vi "LabVIEW Interface MAIN QMH.vi"() -> ()   [LabVIEW 2018]
uses:
  src/geve-serial_config_cluster.ctl
panel:
  out "title":string
  out "Motor Position":dbl
  out "Plateau Pressure":dbl
  out "Pressure":dbl
  out "title1":string="LIVE DATA"
  out "Mixed Signal Graph":T1(graph)
  out "BPM":dbl
  out "PEEP":dbl
  out "Tidal Volume":dbl
  out "IE Ratio":dbl
  out "title 2":string="LIVE DATA"
  out "log":string
  out "INITIALISATION ERROR":bool
  out "HIGH PRESSURE":bool
  out "LOW PRESSURE":bool
  # "LATEST VALUE"
  # "Motor Position"
  # "Plateau Pressure"
  # "Pressure"
  # "POTENTIOMETERS SETTINGS"
  # "BPM"
  # "PEEP"
  # "IE RATIO"
  # "TIDAL VOLUME"
  # "ALARMS"
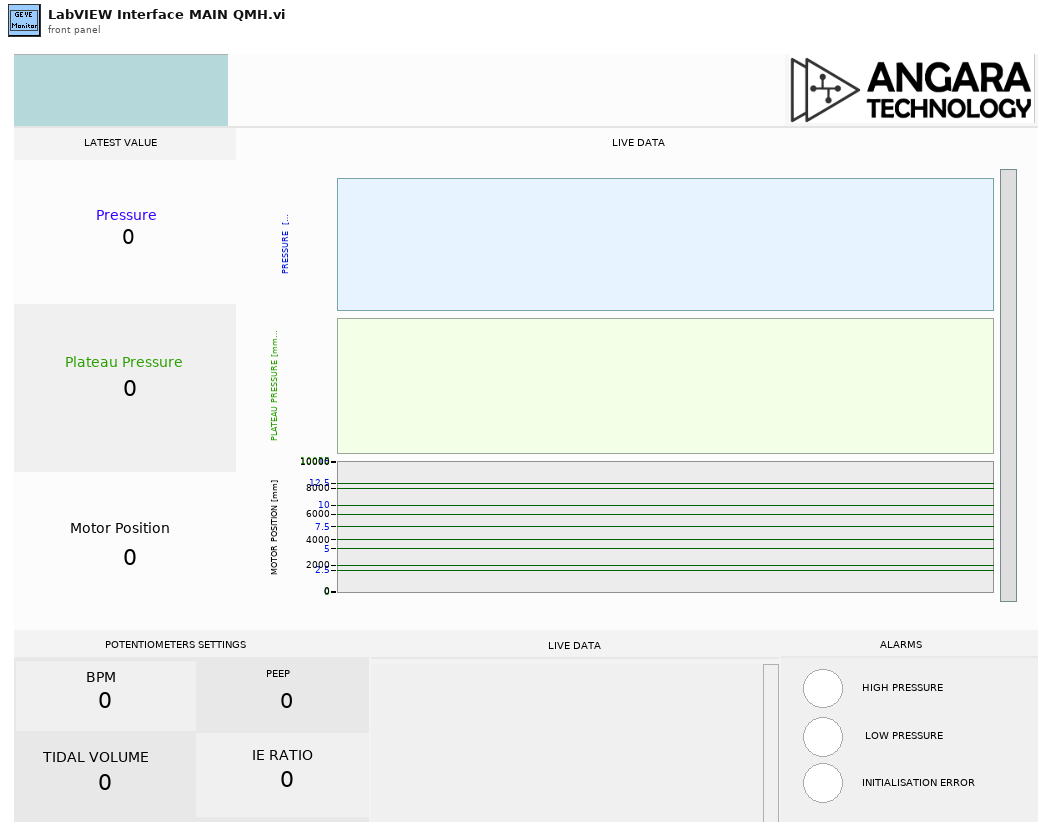
[diagram p1: front panel]
types:
  T1 = cluster{"Time Stamp Array":timestamp[], "Time Stamp Array":dbl[]}[]
  T2 = typedef "geve-runtime_data_cluster.ctl" = cluster{"GEVE Ventilator Monitoring Data":T3, "Serial Port Configuration":T4, "Serial Read Return Count":u32, "Read Buffer":string, "Communication Timeout?":bool, "com-refs":T5}
  T3 = typedef "geve-monitoring_data_cluster.ctl" = cluster{"On/Off":bool, "Error Ack":bool, "bpm":dbl, "VT":dbl, "IE":dbl, "PEEP":dbl, "Pressure":dbl, "Plateau Pressure":dbl, "Motor Position":dbl, "Alarm P High":bool, "Alarm P Low":bool, "Alarm Init":bool}
  T4 = typedef "geve-serial_config_cluster.ctl" = cluster{"timeout (ms)":u32, "VISA resource name":refnum<visa-resource-name>, "baud rate":u32, "max expected byte count":u32}
  T5 = typedef "geve-com_ref_cluster.ctl" = cluster{"msg-self Q":refnum<queue>, "gui stop event":refnum<user-event>}
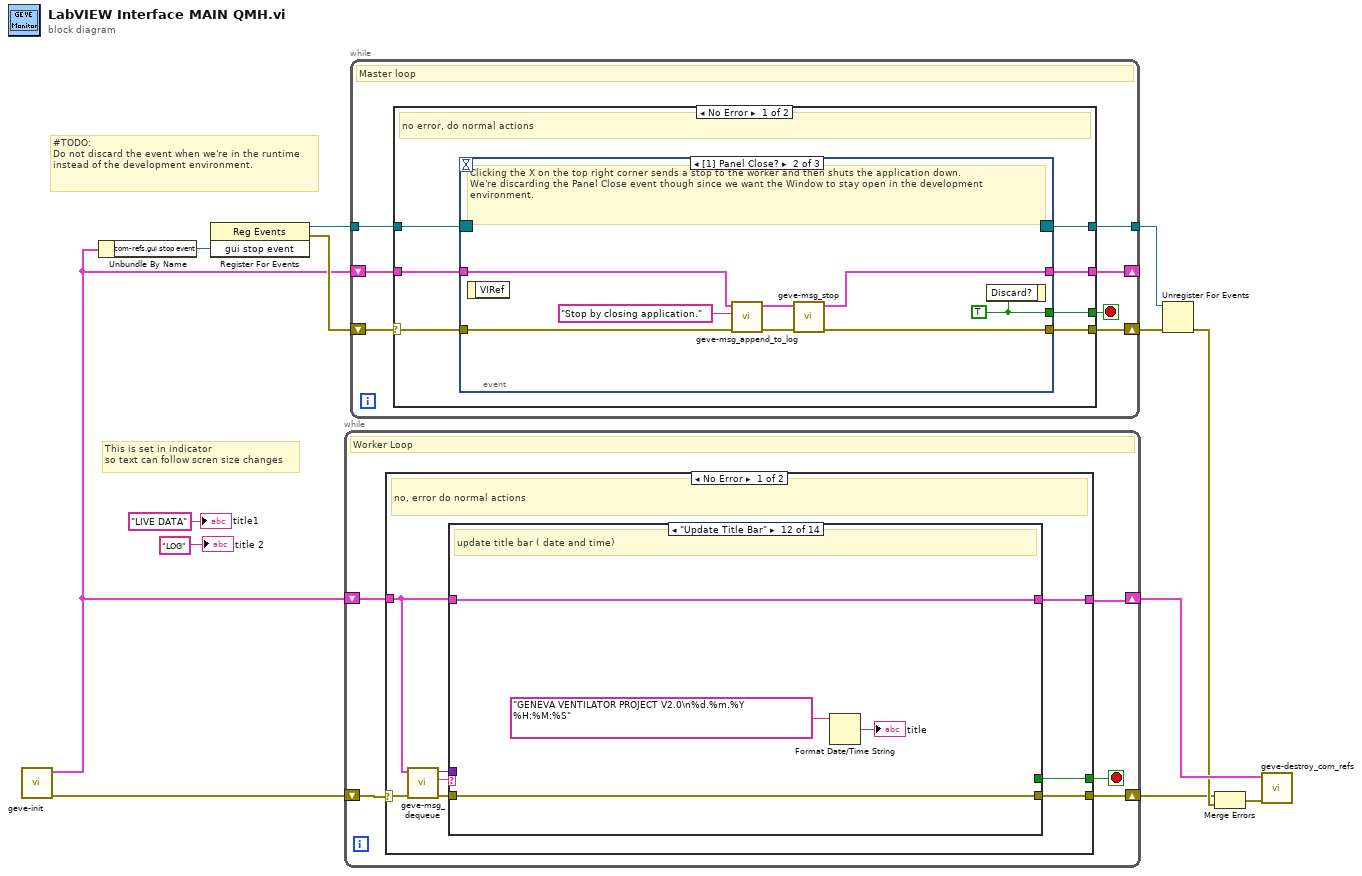
[diagram p0: block diagram]
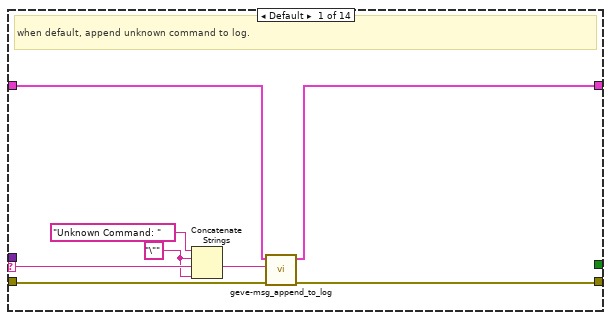
[diagram p2: hidden frame]
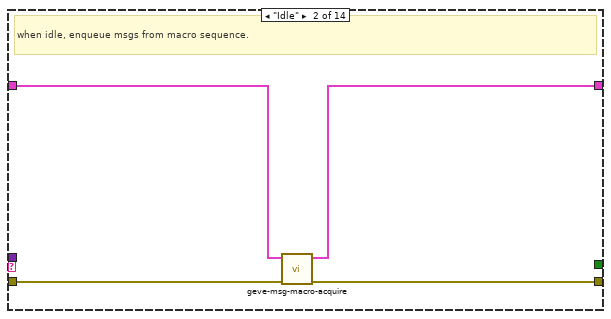
[diagram p3: hidden frame]
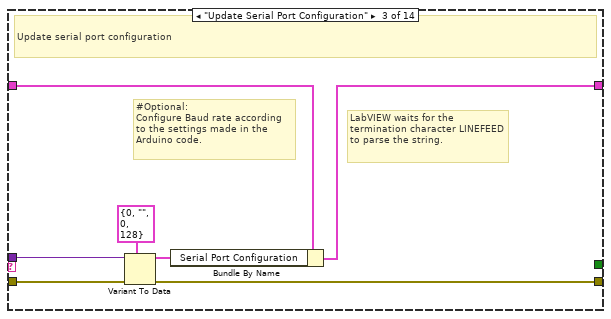
[diagram p4: hidden frame]
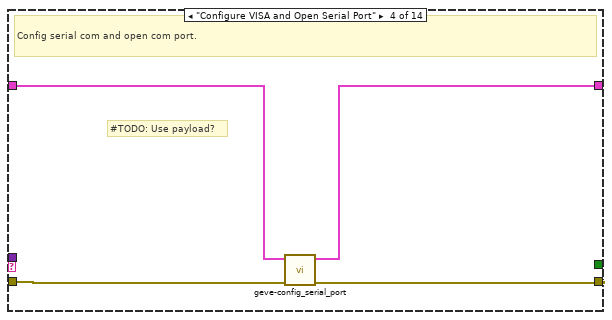
[diagram p5: hidden frame]
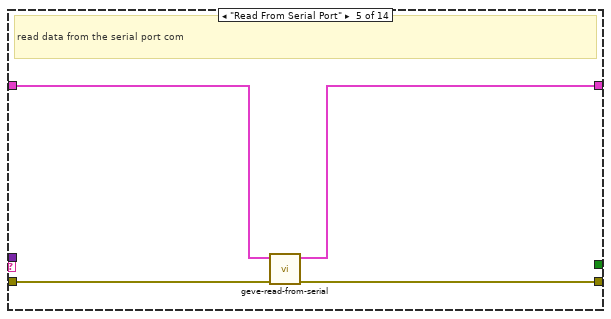
[diagram p6: hidden frame]
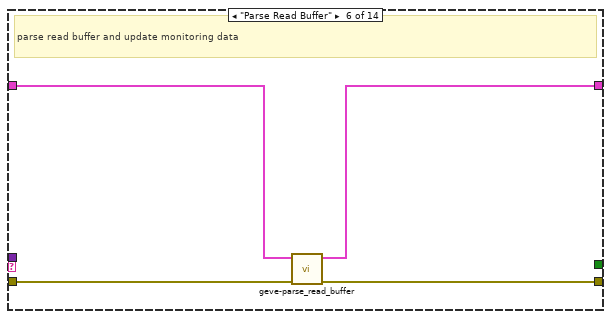
[diagram p7: hidden frame]
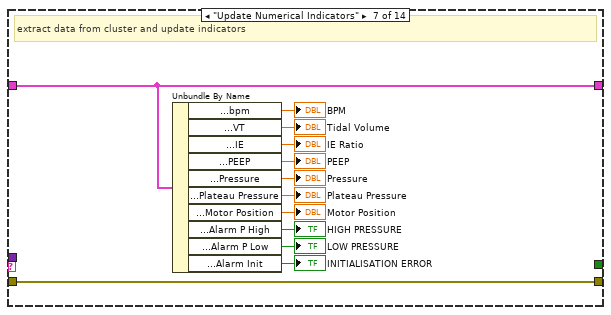
[diagram p8: hidden frame]
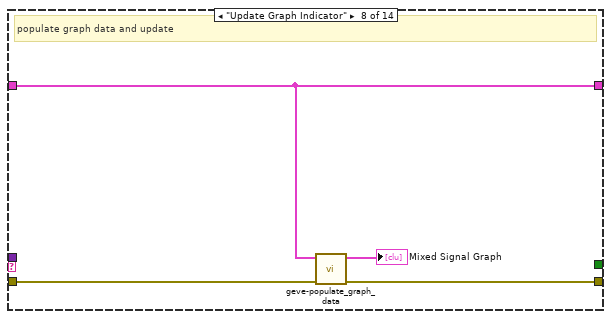
[diagram p9: hidden frame]
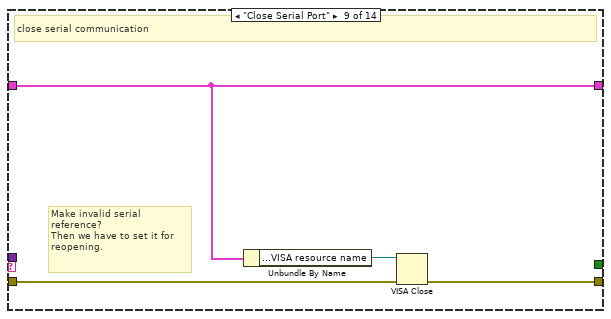
[diagram p10: hidden frame]
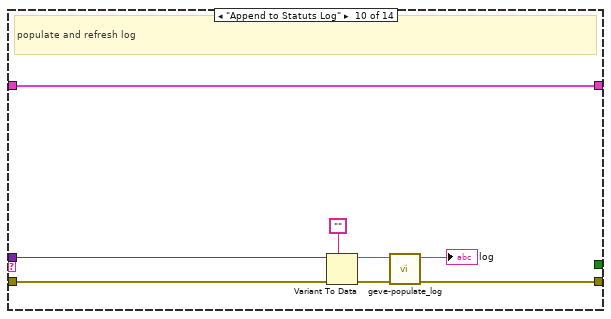
[diagram p11: hidden frame]
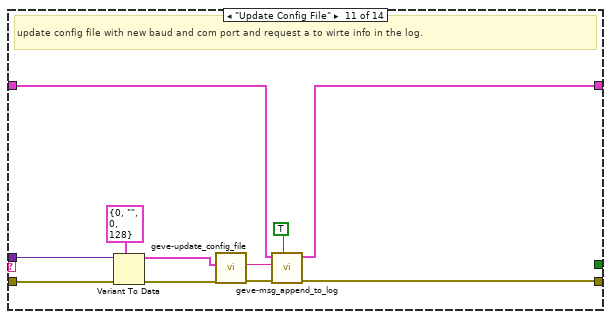
[diagram p12: hidden frame]
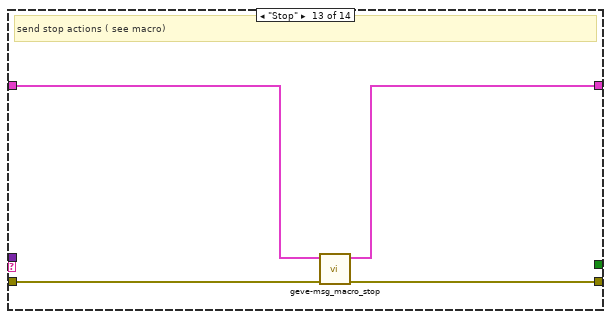
[diagram p13: hidden frame]
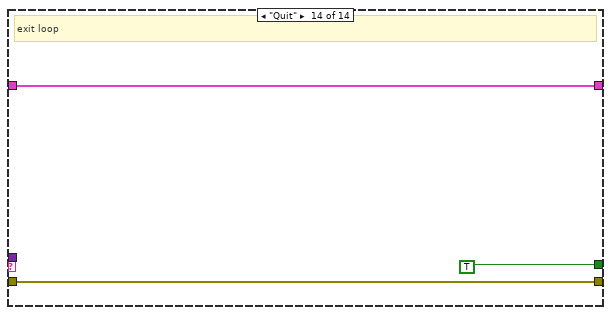
[diagram p14: hidden frame]
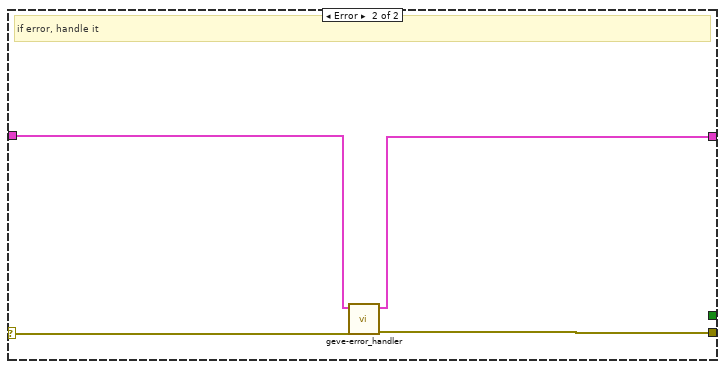
[diagram p15: hidden frame]
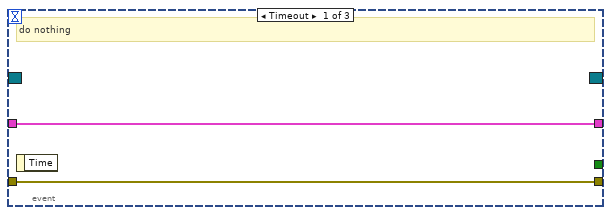
[diagram p16: hidden frame]
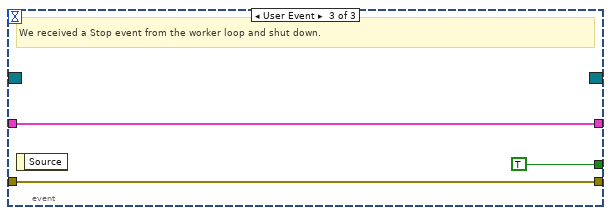
[diagram p17: hidden frame]
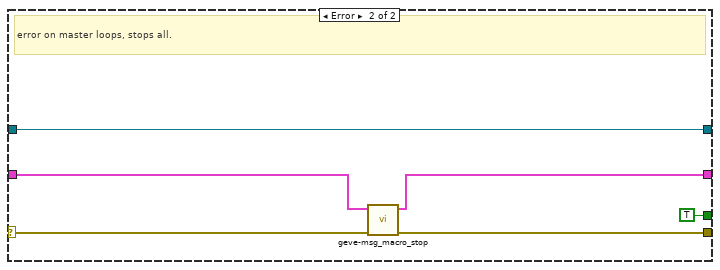
[diagram p18: hidden frame]
diagram:
  # "This is set in indicator\nso text can follow scren size changes"
  # "#TODO:\nDo not discard the event when we're in the runtime instead of the development environment."
  n1 = call "geve-init.vi"() -> ("error out"=w12:errorcluster, "Runtime Data"=w6:T2)  [unwired: 10 in]
  n2 = Unbundle By Name(w6) -> ("com-refs.gui stop event"=w7:refnum<user-event>)
  n3 = register-events(w7) -> (reference out=w11:refnum<event-registration>, error out=w10:errorcluster)  [unwired: 2 in]
  n4 = while {
    shift-right: [w15] -> w13
    shift-left: w6 -> [w17]
    shift-right: [w14] -> w4
    shift-left: w12 -> [w16]
    stop <- w18 stop-if-true
    # "Worker Loop"
    n5 = case shown="No Error" w16 {
      selector: w16 -> [w21 w111]
      tunnel: [w25 _] -> w18
      tunnel: [w24 w110] -> w14
      tunnel: [w23 w108] -> w15
      tunnel: w17 -> [w22 w109]
      frame No Error {
        # "no, error do normal actions"
        n6 = call "geve-msg_dequeue.vi"("error in (no error)"=w21, "Runtime Data"=w22) -> ("error out"=w26:errorcluster, "Command"=w19:string, "Payload"=w20:variant)  [unwired: 7 in]
        n7 = case shown="\"Update Title Bar\"" w19 {
          selector: w19 -> [w34 _ _ _ _ _ _ _ _ _ _ _ _ _]
          tunnel: w20 -> [_ _ w43 _ _ _ _ _ _ w83 w95 _ _ _]
          tunnel: [w30 w37 w39 w46 w50 w56 w69 w70 w76 w79 w87 w100 w103 w107] -> w24
          tunnel: w26 -> [w31 w36 w40 w49 w53 w57 w69 w71 w77 w84 w94 w100 w104 w107]
          tunnel: [w28 w35 w45 w47 w52 w54 w58 w73 w75 w85 w88 w99 w101 w106] -> w23
          tunnel: w22 -> [w29 w38 w44 w48 w51 w55 w58 w73 w75 w85 w89 w99 w102 w106]
          tunnel: [_ _ _ _ _ _ _ _ _ _ _ _ _ TRUE] -> w25
          frame Default {
            w27 = "\"" ("string")
            # "when default, append unknown command to log."
            n8 = Concatenate Strings("Unknown Command: " ("message"), w27, w34, w27) -> (w32:string)
            n9 = call "geve-msg_append_to_log.vi"("error in (no error)"=w31, "Status Message"=w32, "Runtime Data"=w29) -> ("error out"=w30:errorcluster, "Runtime Dataout"=w28:T2)  [unwired: 7 in]
          }
          frame "Idle" {
            # "when idle, enqueue msgs from macro sequence."
            n10 = call "geve-msg-macro-acquire.vi"("error in (no error)"=w36, "Runtime Data"=w38) -> ("error out"=w37:errorcluster, "Runtime Data out"=w35:T2)  [unwired: 8 in]
          }
          frame "Update Serial Port Configuration" {
            # "#Optional:\nConfigure Baud rate according to the settings made in the Arduino code."
            # "LabVIEW waits for the termination character LINEFEED to parse the string."
            # "Update serial port configuration"
            n11 = Variant To Data(error in=w40, type=T4 {"timeout (ms)"=0, "VISA resource name"="", "baud rate"=0, "max expected byte count"=128} ("Serial Port Configuration"), Variant=w43) -> (data=w41:T4, error out=w39:errorcluster)
            n12 = Bundle By Name(cluster=w44, "Serial Port Configuration"=w41) -> (w45:T2)
          }
          frame "Configure VISA and Open Serial Port" {
            # "#TODO: Use payload?"
            # "Config serial com and open com port."
            n13 = call "geve-config_serial_port.vi"("error in (no error)"=w49, "Runtime Data in"=w48) -> ("error out"=w46:errorcluster, "Runtime Data out"=w47:T2)  [unwired: 8 in]
          }
          frame "Read From Serial Port" {
            # "read data from the serial port com"
            n14 = call "geve-read-from-serial.vi"("error in (no error)"=w53, "Runtime Data in"=w51) -> ("error out"=w50:errorcluster, "Runtime Data out"=w52:T2)  [unwired: 8 in]
          }
          frame "Parse Read Buffer" {
            # "parse read buffer and update monitoring data"
            n15 = call "geve-parse_read_buffer.vi"("error in (no error)"=w57, "Runtime Data in"=w55) -> ("error out"=w56:errorcluster, "Runtime Data out"=w54:T2)  [unwired: 8 in]
          }
          frame "Update Numerical Indicators" {
            # "extract data from cluster and update indicators"
            n16 = Unbundle By Name(w58) -> ("GEVE Ventilator Monitoring Data.bpm"=→"BPM":dbl, "GEVE Ventilator Monitoring Data.VT"=→"Tidal Volume":dbl, "GEVE Ventilator Monitoring Data.IE"=→"IE Ratio":dbl, "GEVE Ventilator Monitoring Data.PEEP"=→"PEEP":dbl, "GEVE Ventilator Monitoring Data.Pressure"=→"Pressure":dbl, "GEVE Ventilator Monitoring Data.Plateau Pressure"=→"Plateau Pressure":dbl, "GEVE Ventilator Monitoring Data.Motor Position"=→"Motor Position":dbl, "GEVE Ventilator Monitoring Data.Alarm P High"=→"HIGH PRESSURE":bool, "GEVE Ventilator Monitoring Data.Alarm P Low"=→"LOW PRESSURE":bool, "GEVE Ventilator Monitoring Data.Alarm Init"=→"INITIALISATION ERROR":bool)
          }
          frame "Update Graph Indicator" {
            # "populate graph data and update"
            n17 = call "geve-populate_graph_data.vi"("error in (no error)"=w71, "Runtime Data"=w73) -> ("error out"=w70:errorcluster, "graph data"=→"Mixed Signal Graph":T1)  [unwired: 8 in]
          }
          frame "Close Serial Port" {
            # "Make invalid serial reference?\nThen we have to set it for reopening."
            # "close serial communication"
            n18 = Unbundle By Name(w75) -> ("Serial Port Configuration.VISA resource name"=w74:refnum<visa-resource-name>)
            n19 = VISA Close(VISA resource name=w74, error in (no error)=w77) -> (error out=w76:errorcluster)
          }
          frame "Append to Statuts Log" {
            # "populate and refresh log"
            n20 = Variant To Data(error in=w84, type="", Variant=w83) -> (data=w81:string, error out=w80:errorcluster)
            n21 = call "geve-populate_log.vi"("error in (no error)"=w80, "String in"=w81) -> ("error out"=w79:errorcluster, "log out"=→"log":string)  [unwired: 8 in]
          }
          frame "Update Config File" {
            # "update config file with new baud and com port and request a to wirte info in the log."
            n22 = Variant To Data(error in=w94, type=T4 {"timeout (ms)"=0, "VISA resource name"="", "baud rate"=0, "max expected byte count"=128} ("Serial Port Configuration"), Variant=w95) -> (data=w92:T4, error out=w93:errorcluster)
            n23 = call "geve-update_config_file.vi"("error in (no error)"=w93, "Serial Port Configuration"=w92) -> ("error out"=w90:errorcluster, "info"=w91:string)  [unwired: 7 in, 1 out]
            n24 = call "geve-msg_append_to_log.vi"("Priority"=TRUE, "error in (no error)"=w90, "Status Message"=w91, "Runtime Data"=w89) -> ("error out"=w87:errorcluster, "Runtime Dataout"=w88:T2)  [unwired: 6 in]
          }
          frame "Update Title Bar" {
            # "update title bar ( date and time)"
            n25 = Format Date/Time String(time format string (%c)="GENEVA VENTILATOR PROJECT V2.0\n%d.%m.%Y      %H:%M:%S") -> (date/time string=→"title":string)  [unwired: 2 in]
          }
          frame "Stop" {
            # "send stop actions ( see macro)"
            n26 = call "geve-msg_macro_stop.vi"("error in (no error)"=w104, "Runtime Data"=w102) -> ("error out"=w103:errorcluster, "Runtime Data out"=w101:T2)  [unwired: 8 in]
          }
          frame "Quit" {
            # "exit loop"
          }
        }
      }
      frame Error {
        # "if error, handle it"
        n27 = call "geve-error_handler.vi"("error in (no error)"=w111, "Runtime Data in"=w109) -> ("error out"=w110:errorcluster, "Runtime Data out"=w108:T2)  [unwired: 8 in]
      }
    }
  }
  n28 = while {
    tunnel: w11 -> [w116]
    tunnel: [w114] -> w8
    shift-right: [w113] -> _
    shift-left: w6 -> [w117]
    shift-right: [w115] -> w9
    shift-left: w10 -> [w112]
    stop <- w118 stop-if-true
    # "Master loop"
    n29 = case shown="No Error" w112 {
      selector: w112 -> [w119 w140]
      tunnel: [w125 TRUE ("NewVal")] -> w118
      tunnel: w117 -> [w124 w142]
      tunnel: w116 -> [w123 w144]
      tunnel: [w122 w139] -> w115
      tunnel: [w121 w144] -> w114
      tunnel: [w120 w141] -> w113
      frame No Error {
        # "no error, do normal actions"
        n30 = event shown="[1] Panel Close?" {
          selector: w123 -> [_ _ _]
          dyn-events: [_ _ _] -> w121
          timeout: _ -> [_ _ _]
          tunnel: [_ w135 TRUE ("NewVal")] -> w125
          tunnel: w124 -> [w126 w129 w136]
          tunnel: w119 -> [w127 w131 w137]
          tunnel: [w127 w132 w137] -> w122
          tunnel: [w126 w128 w136] -> w120
          event Timeout {
            # "do nothing"
            n31 = event-data() -> ()  [unwired: 1 in, 1 out]
          }
          event Panel Close? {
            w135 = TRUE ("NewVal")
            # "Clicking the X on the top right corner sends a stop to the worker and then shuts the application down.\nWe're discarding the Panel Close event though since we want the Window to stay open in the development environment."
            n32 = event-data() -> ()  [unwired: 1 in, 1 out]
            n33 = call "geve-msg_append_to_log.vi"("error in (no error)"=w131, "Status Message"="Stop by closing application.", "Runtime Data"=w129) -> ("error out"=w133:errorcluster, "Runtime Dataout"=w130:T2)  [unwired: 7 in]
            n34 = call "geve-msg_stop.vi"("error in (no error)"=w133, "Runtime Data"=w130) -> ("error out"=w132:errorcluster, "Runtime Data out"=w128:T2)  [unwired: 8 in]
            n35 = event-data("Discard?"=w135) -> ()  [unwired: 1 in, 1 out]
          }
          event User Event {
            # "We received a Stop event from the worker loop and shut down."
            n36 = event-data() -> ()  [unwired: 1 in, 1 out]
          }
        }
      }
      frame Error {
        # "error on master loops, stops all."
        n37 = call "geve-msg_macro_stop.vi"("error in (no error)"=w140, "Runtime Data"=w142) -> ("error out"=w139:errorcluster, "Runtime Data out"=w141:T2)  [unwired: 8 in]
      }
    }
  }
  n38 = Unregister For Events(event registration refnum=w8, error in=w9) -> (error out=w5:errorcluster)
  n39 = Merge Errors(w4, w5) -> (w3:errorcluster)
  n40 = call "geve-destroy_com_refs.vi"("error in (no error)"=w3, "Runtime Data"=w13) -> ()  [unwired: 10 in]
  "title1" <- "LIVE DATA" ("String")
  "title 2" <- "LOG" ("String")
